vi "SendStopSaving.vi"(8 "error in (no error)":errorcluster, 11 "Application Data":T1) -> (0 "error out":errorcluster)   [LabVIEW 2019]
uses:
  Typedefs/#cluster_ApplicationData.ctl
  Typedefs/Acquisition Thread/#cluster_AcqQueueData.ctl
  Typedefs/Acquisition Thread/#enum_AcquisitionTask.ctl
  Typedefs/Saving Thread/#cluster_SavingQueueData.ctl
  Typedefs/Saving Thread/#enum_SavingTask.ctl
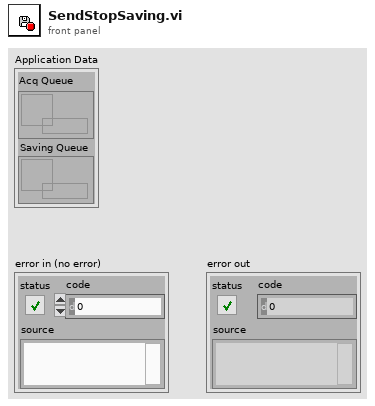
[diagram p1: front panel]
types:
  T1 = typedef "#cluster_ApplicationData.ctl" = cluster{"Acq Queue":refnum<queue>, "Saving Queue":refnum<queue>}
  T2 = typedef "#cluster_SavingQueueData.ctl" = cluster{"Task":T3, "Data":variant}
  T3 = typedef "#enum_SavingTask.ctl" = enum16{"Set directory", "Save", "Stop", "Close"}
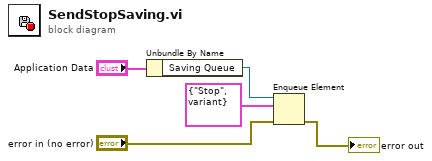
[diagram p0: block diagram]
diagram:
  n1 = Unbundle By Name("Application Data") -> ("Saving Queue"=w4:refnum<queue>)
  n2 = Enqueue Element(queue=w4, element=T2 {"Task"=enum."Stop", "Data"=variant}, error in (no error)="error in (no error)") -> (error out=→"error out":errorcluster)  [unwired: 1 in, 2 out]
